vi "RM interrupt timing GUID Lookup.vi"() -> ()   [LabVIEW 2014, in "RM interrupt timing Custom Device.lvlib"]
doc: "Use this Global VI to access the GUIDs assigned to the page resources of the Custom Device."
uses:
  RM interrupt timing Custom Device.lvlib
panel:
  in  "4":string="ef76cc62-07d1-45ce-bf79-428e76fe87ec"
  in  "3":string="4e118a9d-169a-4916-861a-6b7bd16585a4"
  in  "2":string="91250044-a79c-408f-bd0b-9298a06faf04"
  in  "1":string="aaa2a357-c104-40f6-8bbc-9b1347fa38b7"
  in  "Custom Device":string="2bb7d41b-e389-40ed-82da-8f995ad3e21b"
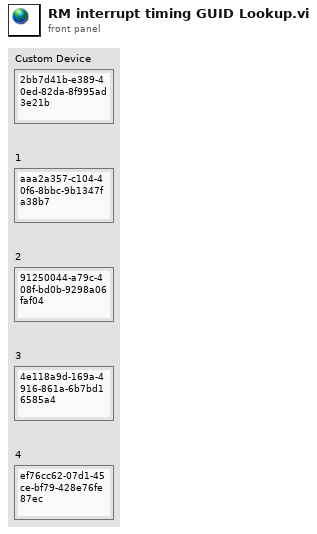
[diagram p1: front panel]
diagram:
